vi "fake tool arrays.vi"(8 "boolarray":bool[](array[boolean]), 9 "intarray":i32[](array[numeric]), 10 "doublearray":dbl[](array[numeric]), 11 "stringarray":string[](array[string])) -> (3 "result string":string)   [LabVIEW 2020, in "MCP Server tests.lvlib"]
doc: "Fake tool to test if array datatypes are parsed correctly."
uses:
  MCP Server tests.lvlib
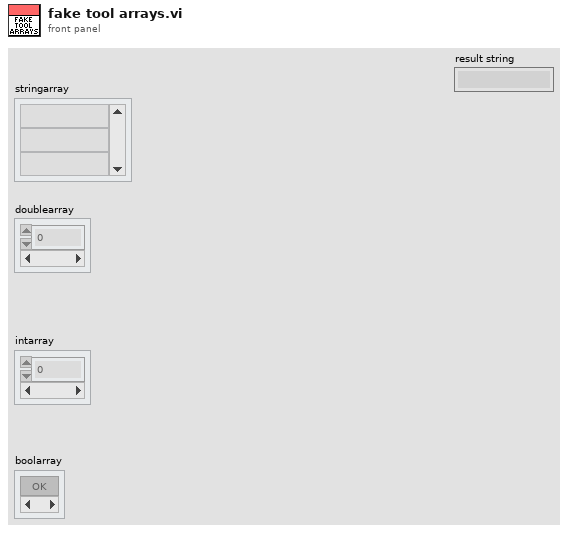
[diagram p1: front panel]
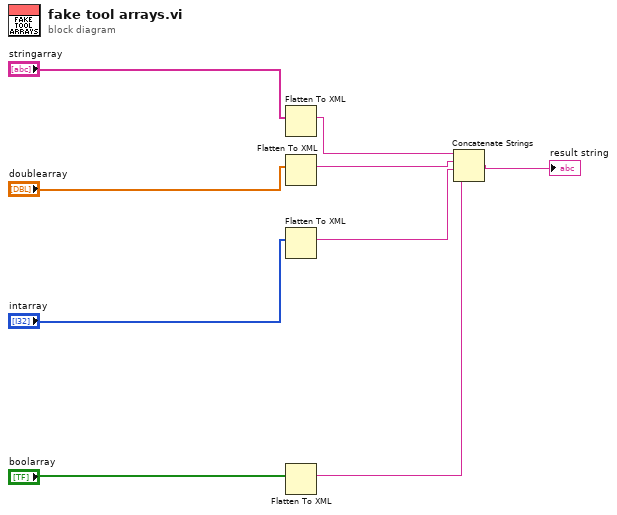
[diagram p0: block diagram]
diagram:
  n1 = Flatten To XML(6:"stringarray") -> (2:w5:string)
  n2 = Flatten To XML(6:"doublearray") -> (2:w4:string)
  n3 = Flatten To XML(6:"intarray") -> (2:w3:string)
  n4 = Flatten To XML(6:"boolarray") -> (2:w2:string)
  n5 = Concatenate Strings(w5, w4, w3, w2) -> (→"result string":string)
